vi "Compute Linear Phasor Combination.vi"(4 "Prefactor 2":dbl, 5 "Lifetime 2":dbl[unit], 6 "Prefactor 1":dbl, 7 "Lifetime 1":dbl[unit], 9 "Prefactor Type":enum32{"Exp. Amplitude", "Intensity Fraction"}(radio), 10 "Phasor 2":T1, 11 "Phasor 1":T1) -> (1 "f2":dbl, 2 "f1":dbl, 3 "Phasor (g, s) out":T1)   [LabVIEW 2021, in "Phasor.lvlib"]
uses:
  Phasor (g, s).ctl
  Phasor.lvlib
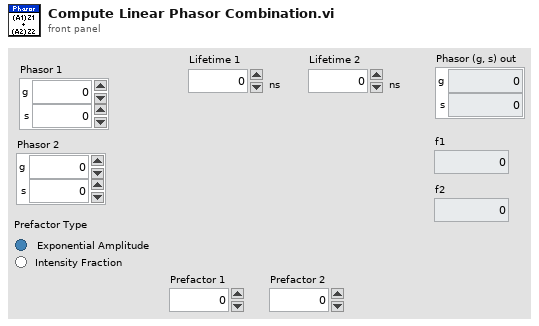
[diagram p1: front panel]
types:
  T1 = typedef "Phasor.lvlib/Phasor (g, s).ctl" = cluster{"g":dbl, "s":dbl}
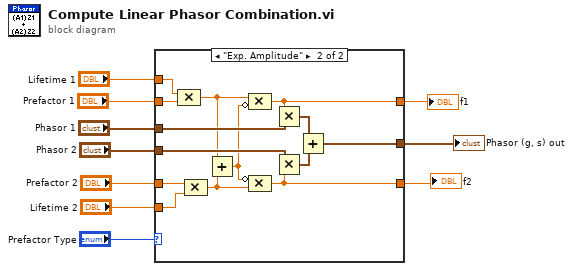
[diagram p0: block diagram]
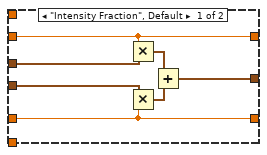
[diagram p2: hidden frame]
diagram:
  n1 = case shown="\"Exp. Amplitude\"" "Prefactor Type" {
    tunnel: [w13 w27] -> w10
    tunnel: "Phasor 2" -> [w17 w31]
    tunnel: "Phasor 1" -> [w16 w30]
    tunnel: "Prefactor 2" -> [w11 w26]
    tunnel: "Prefactor 1" -> [w12 w25]
    tunnel: "Lifetime 1" -> [_ w24]
    tunnel: "Lifetime 2" -> [_ w23]
    tunnel: [w12 w19] -> w2
    tunnel: [w11 w18] -> w1
    frame "Intensity Fraction", Default {
      n2 = Multiply(x=w12, y=w16) -> (x*y=w15:T1)
      n3 = Multiply(x=w17, y=w11) -> (x*y=w14:T1)
      n4 = Add(x=w15, y=w14) -> (x+y=w13:T1)
    }
    frame "Exp. Amplitude" {
      n5 = Compound Arithmetic op=MULTIPLY(w24, w25) -> (w21:dbl[unit])
      n6 = Compound Arithmetic op=MULTIPLY(w26, w23) -> (w22:dbl[unit])
      n7 = Add(x=w21, y=w22) -> (x+y=w20:dbl[unit])
      n8 = Compound Arithmetic op=MULTIPLY(w21, invert w20) -> (w19:dbl)
      n9 = Compound Arithmetic op=MULTIPLY(invert w20, w22) -> (w18:dbl)
      n10 = Multiply(x=w19, y=w30) -> (x*y=w29:T1)
      n11 = Multiply(x=w31, y=w18) -> (x*y=w28:T1)
      n12 = Add(x=w29, y=w28) -> (x+y=w27:T1)
    }
  }
  "Phasor (g, s) out" <- w10
  "f1" <- w2
  "f2" <- w1
